vi "Write TopRef.vi"(8 "error in (no error)":errorcluster, 10 "TopRef":T1, 11 "UIActorTop2 in":refnum<class "CheckPasswordUI.lvclass">) -> (0 "error out":errorcluster, 3 "UIActorTop2 out":refnum<class "CheckPasswordUI.lvclass">)   [LabVIEW 2021, in "CheckPasswordUI.lvclass"]
uses:
  CheckPasswordUI.lvclass
  TopRef.ctl
  CheckPasswordUI.lvclass/CheckPasswordUI.ctl
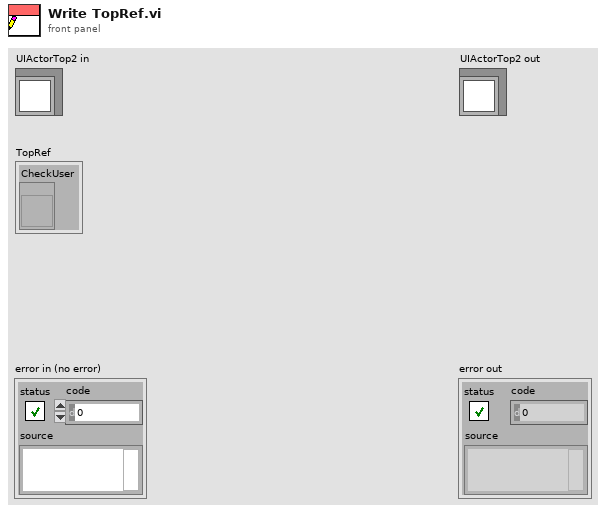
[diagram p1: front panel]
types:
  T1 = typedef "CheckPasswordUI.lvclass/TopRef.ctl" = cluster{"CheckUser":refnum<vi>}
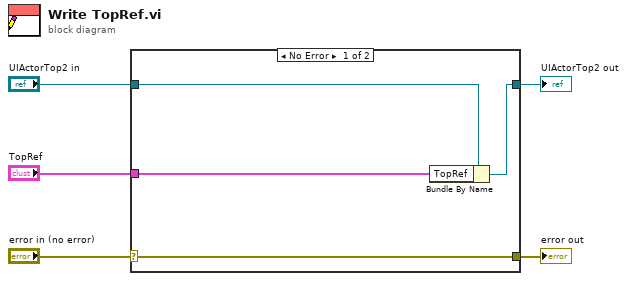
[diagram p0: block diagram]
diagram:
  n1 = case shown="No Error" "error in (no error)" {
    selector: "error in (no error)" -> [w9 w10]
    tunnel: [w9 w10] -> w4
    tunnel: [w7 w11] -> w2
    tunnel: "UIActorTop2 in" -> [w8 w11]
    tunnel: "TopRef" -> [w6 _]
    frame No Error {
      n2 = Bundle By Name(cluster=w8, "TopRef"=w6) -> (w7:refnum<class "CheckPasswordUI.lvclass">)
    }
    frame Error {
    }
  }
  "error out" <- w4
  "UIActorTop2 out" <- w2
